vi "获取单元格区域.vi"(1 "单元格区域":T1={"起始列"="A", "起始行"=1, "大小"=[]} {"大小" min=1 max=1048576; "起始行" min=1 max=1048576}) -> (0 "单元格区域":string)   [LabVIEW 2021, in "OperateExcel.lvlib"]
uses:
  OperateExcel.lvlib
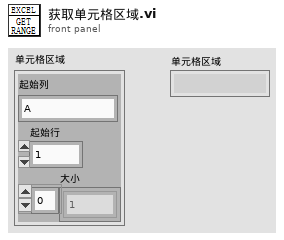
[diagram p1: front panel]
types:
  T1 = typedef "OperateExcel.lvlib/单元格区域.ctl" = cluster{"起始列":string, "起始行":u32, "大小":u32[]}
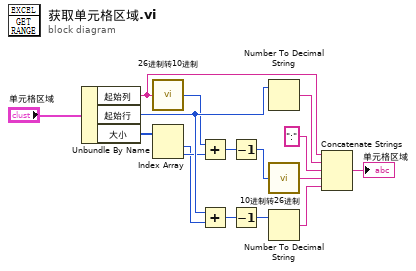
[diagram p0: block diagram]
diagram:
  n1 = Unbundle By Name("单元格区域") -> ("起始列"=w8:string, "起始行"=w9:u32, "大小"=w2:u32[])
  n2 = call "26进制转10进制.vi"("26进制"=w8) -> ("十进制"=w6:u16)
  n3 = Index Array(array=w2) -> (element #1=w3:u32, element #2=w7:u32)  [unwired: 2 in]
  n4 = Add(x=w6, y=w7) -> (x+y=w5:u32)
  n5 = Add(x=w9, y=w3) -> (x+y=w4:u32)
  n6 = Decrement(x=w5) -> (x-1=w12:u32)
  n7 = Decrement(x=w4) -> (x-1=w14:u32)
  n8 = Number To Decimal String(number=w9) -> (decimal integer string=w10:string)  [unwired: 1 in]
  n9 = call "10进制转26进制.vi"("十进制"=w12) -> ("26进制"=w13:string)
  n10 = Number To Decimal String(number=w14) -> (decimal integer string=w15:string)  [unwired: 1 in]
  n11 = Concatenate Strings(w8, w10, ":" ("字符串"), w13, w15) -> (→"单元格区域":string)
